vi "propagation_lbl.vi"(0 "HAS analyzer paths":T3={"Haso configuration"=path "C:/Program Files (x86)/Imagine Optic/Configuration Files/HASO4_first_7564.dat", "HAS folder"=path "N:/data/Y2019/12-Dec/19_1212/analysis/Scan026/HASOCopyAA", "subtract ref has"=FALSE, "Slopes file to subtract"=path "Z:/data/TestStand/Y2021/03-Mar/21_0303/scans/Scan006/TapeHASOCopy/Scan006_TapeHASOCopy_019.has", "Slopes file name"=path "D:/Server/10_Software/LabVIEW VIs/ImagineOptic/s35test_new.has"}, 1 "filter":T6, 2 "source wavelength [nm] (if not in has file)":dbl=800.0 format="%#_13g", 5 "Pupil":T1, 7 "Perfect lens":T10={"lens_m"=0.0, "KeepCurvature"=TRUE}, 9 "defocus":sgl, 11 "error in (no error)":errorcluster, 12 "filter":bool) -> (3 "StatisticsData":T5, 4 "PSF values":sgl[][](graph), 6 "PSF_Dimensions_um":T7, 8 "radius_mm":sgl, 10 "Wavefront (micron)":sgl[][](graph), 14 "parameters":T4, 15 "error out":errorcluster)   [LabVIEW 2020]
uses:
  WaveKit/Controls/StatisticsData.ctl
  WaveKit/Controls/SlopesPostProcessorList - Add lens.ctl
  WaveKit/Controls/General dimensions definition.ctl
  WaveKit/Controls/Point2D.ctl
  WaveKit/Controls/Point2Df.ctl
  WaveKit/Controls/HAS File information.ctl
  WaveKit/Controls/SlopesPostProcessorList - Filter.ctl
  HAS analyzer paths.ctl
  pupil ajg.ctl
  WaveKit/Classes/HasoSlopes/HasoSlopes.lvclass
  WaveKit/Classes/Pupil/Pupil.lvclass
  WaveKit/Classes/HasoField/HasoField.lvclass
  WaveKit/Classes/SurfaceFloat/SurfaceFloat.lvclass
  WaveKit/Classes/Phase/Phase.lvclass
  WaveKit/Classes/HasoData/HasoData.lvclass
  WaveKit/Classes/ComputePhaseSet/ComputePhaseSet.lvclass
panel:
  out "Zernike pupil":i32[][](graph)
  in  "PSF":bool
  out "HAS file information":T9 {"Source wavelength (nm)" format="%#_2g"}
  out "Dimension_um":T7
  in  "param":T11={"null_phase"=FALSE, "flat_intensity"=TRUE}
  out "PSF Statistics":T5={"PV"=1374189.0, "RMS"=17526034.0, "Max"=17526036.0, "Min"=1.2032529}
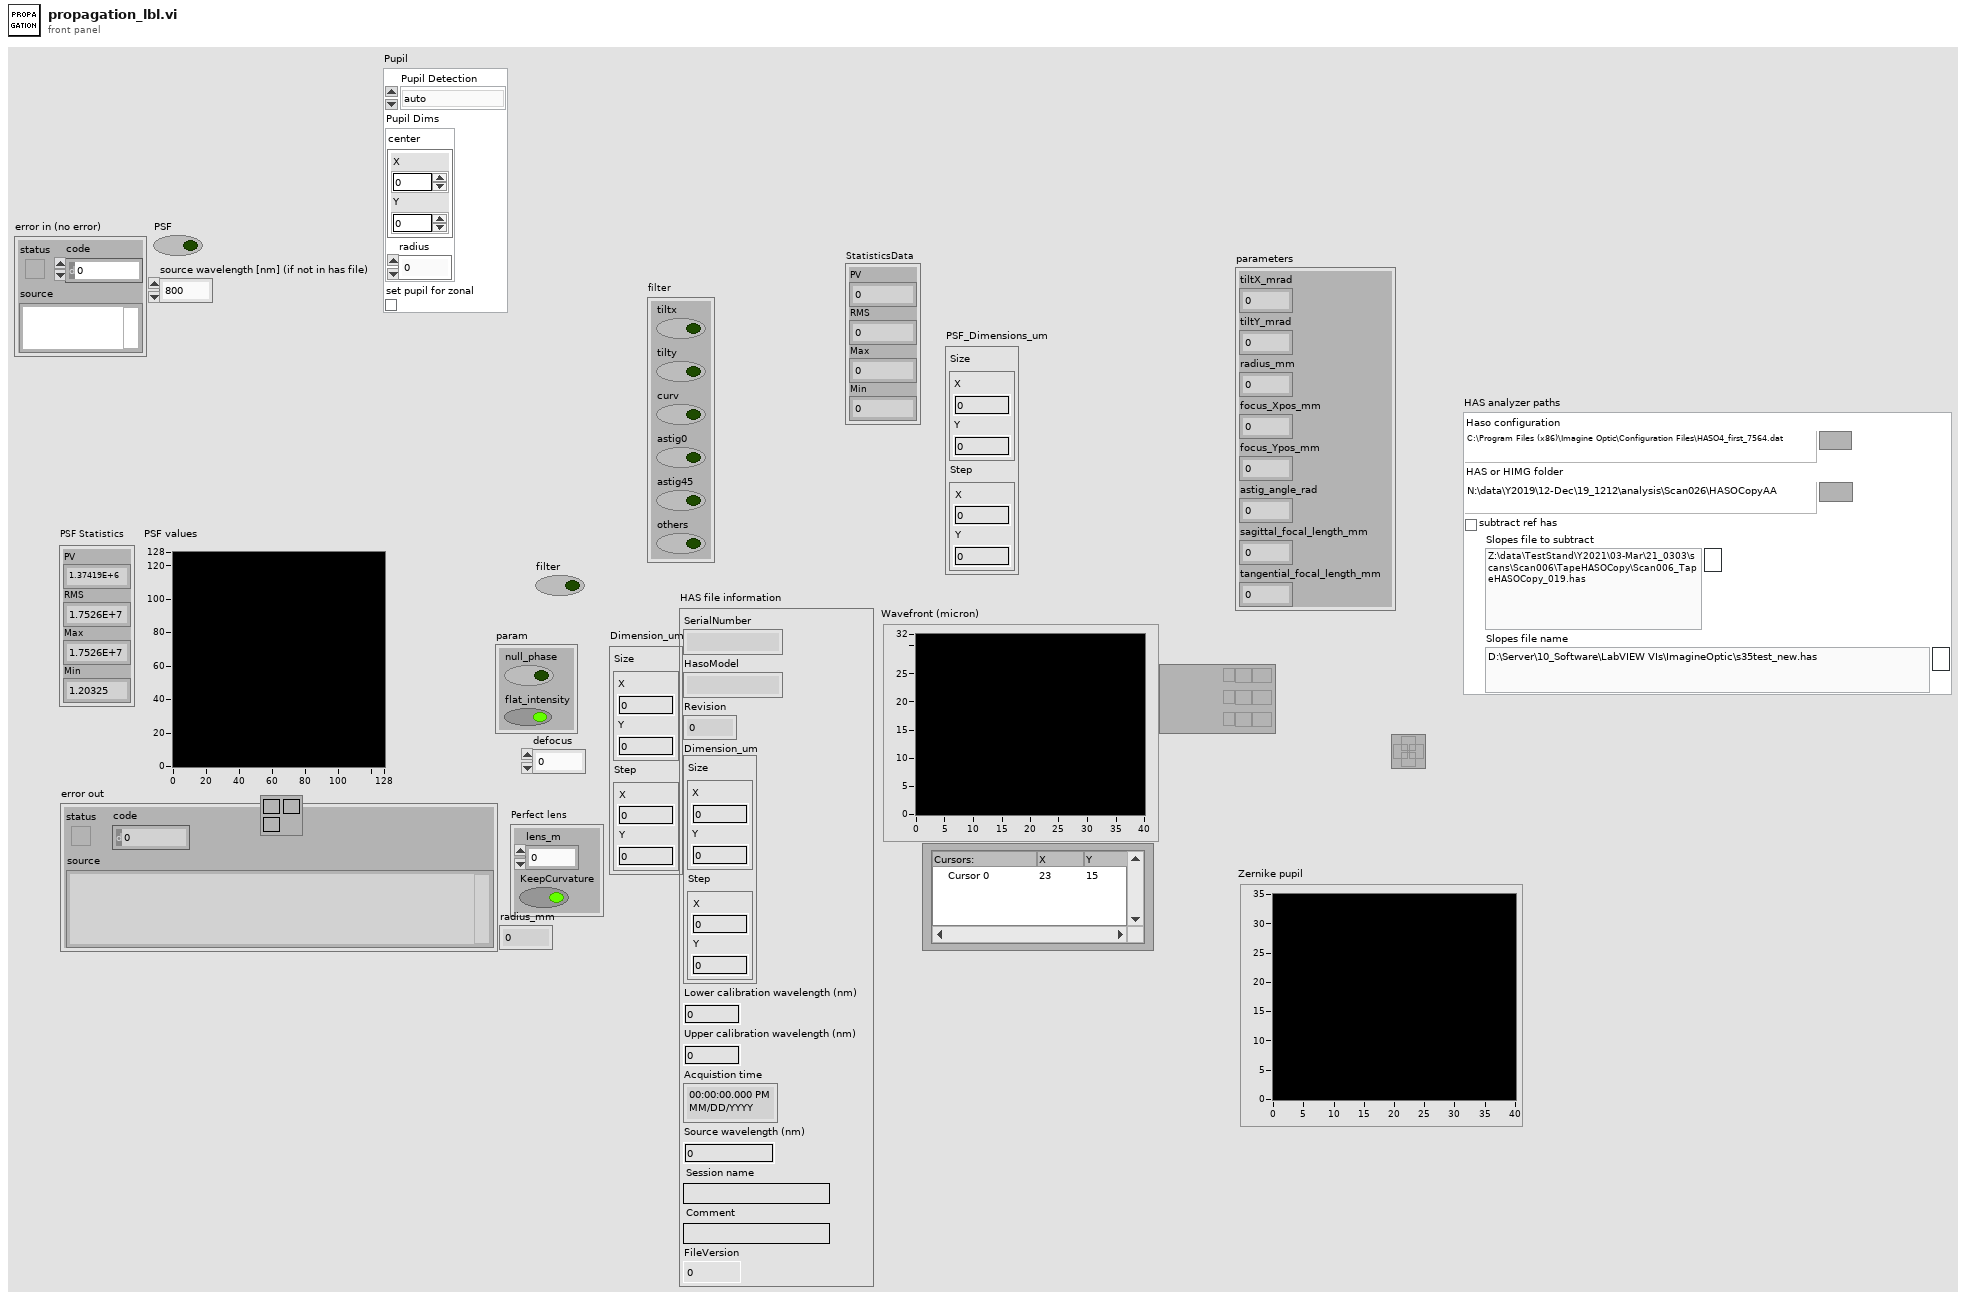
[diagram p1: front panel]
types:
  T1 = typedef "pupil ajg.ctl" = cluster{"Pupil Detection":enum16{"auto", "auto 1st shot only", "manual"}, "Pupil Dims":cluster{"center":T2, "radius":sgl}, "set pupil for zonal":bool}
  T2 = typedef "Point2Df.ctl" = cluster{"X":sgl, "Y":sgl}
  T3 = typedef "HAS analyzer paths.ctl" = cluster{"Haso configuration":path, "HAS folder":path, "subtract ref has":bool, "Slopes file to subtract":path, "Slopes file name":path}
  T4 = cluster{"tiltX_mrad":sgl, "tiltY_mrad":dbl, "radius_mm":sgl, "focus_Xpos_mm":sgl, "focus_Ypos_mm":sgl, "astig_angle_rad":sgl, "sagittal_focal_length_mm":sgl, "tangential_focal_length_mm":sgl}
  T5 = typedef "StatisticsData.ctl" = cluster{"PV":sgl, "RMS":dbl, "Max":sgl, "Min":sgl}
  T6 = typedef "SlopesPostProcessorList - Filter.ctl" = cluster{"tiltx":bool, "tilty":bool, "curv":bool, "astig0":bool, "astig45":bool, "others":bool}
  T7 = typedef "General dimensions definition.ctl" = cluster{"Size":T8, "Step":T2}
  T8 = typedef "Point2D.ctl" = cluster{"X":u32, "Y":u32}
  T9 = typedef "HAS File information.ctl" = cluster{"SerialNumber":string, "HasoModel":string, "Revision":u32, "Dimension_um":T7, "Lower calibration wavelength (nm)":dbl, "Upper calibration wavelength (nm)":dbl, "Acquistion time":timestamp, "Source wavelength (nm)":dbl, "Session name":string, "Comment":string, "FileVersion":i32}
  T10 = typedef "SlopesPostProcessorList - Add lens.ctl" = cluster{"lens_m":sgl, "KeepCurvature":bool}
  T11 = cluster{"null_phase":bool, "flat_intensity":bool}
  T12 = typedef "DataHaso acquisition information.ctl" = cluster{"HASO information":T13, "Acquisition information":T14, "SLOPES ENGINE information":T18, "Source wavelength (nm)":dbl, "FillPercent_%":dbl, "session_name":string}
  T13 = typedef "HASO information.ctl" = cluster{"HASO serial number":string, "HASO model":string, "Lower calibration wavelength (nm)":dbl, "Upper calibration wavelength (nm)":dbl, "Revision":i32}
  T14 = typedef "Image information.ctl" = cluster{"Image general information":T15, "Acquisition information":T16, "Number of pixels":T8, "Number of bits":T17}
  T15 = typedef "Image general information.ctl" = cluster{"Camera serial number":string, "Smearing removed":bool, "Background image removed":bool, "Time Stamp":timestamp, "Comment":string, "Camera_MAX_Level":i32}
  T16 = typedef "Image acquisition information.ctl" = cluster{"Exposure duration (us)":i32, "Exposure duration specified (us)":i32, "Gain":sgl, "Number of summed images":i32, "Trigger type":string}
  T17 = typedef "Data alignment enum.ctl" = enum16{"8", "16", "32"}
  T18 = typedef "SlopesEngineSetup.ctl" = cluster{"Start sub-aperture":T8, "Pupil average":dbl, "AutoStartSub-aperture":bool}
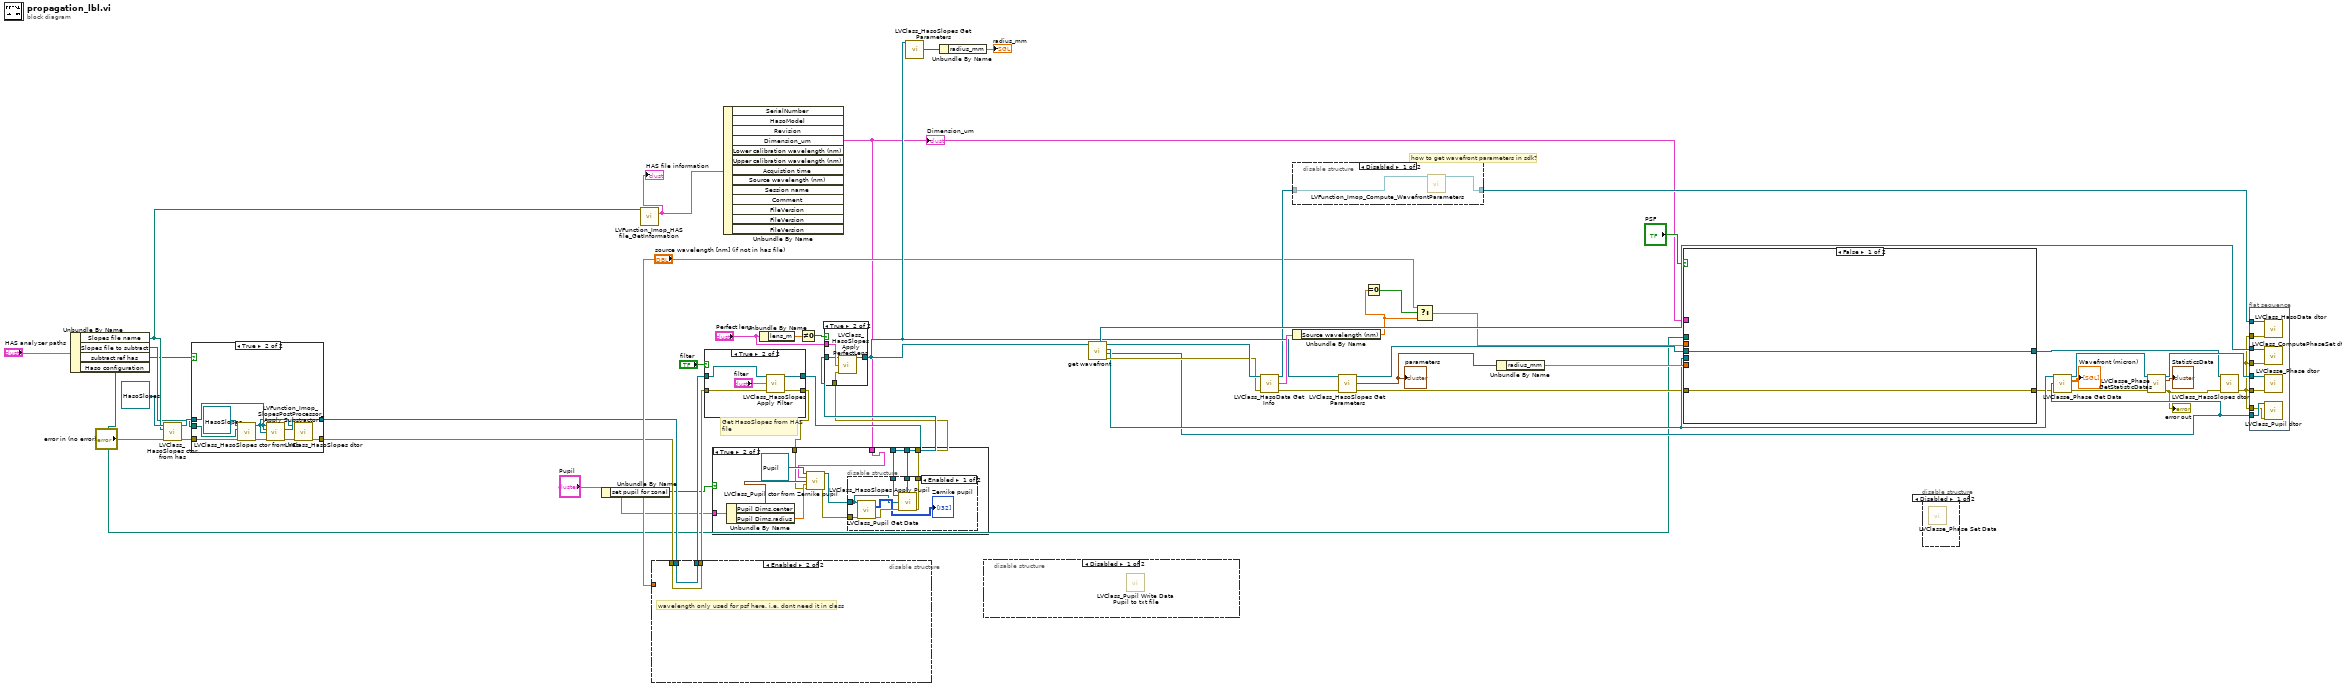
[diagram p0: block diagram]
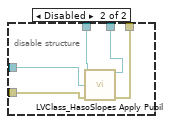
[diagram p3: hidden frame]
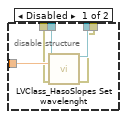
[diagram p6: hidden frame]
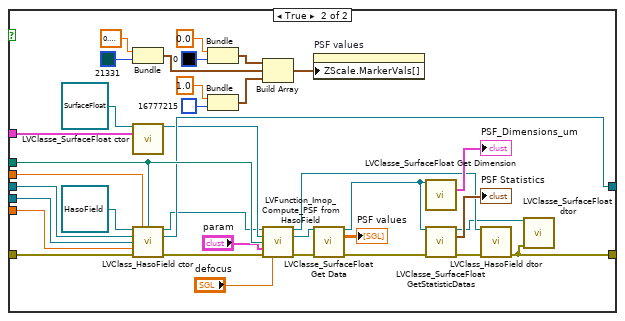
[diagram p7: hidden frame]
diagram:
  # "how to get wavefront parameters in sdk?"
  # "Get HasoSlopes from HAS file"
  n1 = Unbundle By Name("HAS analyzer paths") -> ("Slopes file name"=w10:path, "Slopes file to subtract"=w9:path, "subtract ref has"=w8:bool, "Haso configuration"=w11:path)
  n2 = call "LVClass_HasoSlopes ctor from has.vi"("HasoSlopes (const)"=refnum<class "HasoSlopes.lvclass"> refnum ("HasoSlopes in"), ".has path"=w10, "error in (no error)"="error in (no error)") -> ("HasoSlopes (new)"=w16:refnum<class "HasoSlopes.lvclass">, "error out"=w15:errorcluster)  [unwired: 11 in]
  n3 = case shown="True" w8 {
    tunnel: w9 -> [_ w66]
    tunnel: [w57 w65] -> w17
    tunnel: w16 -> [w57 w64]
    tunnel: w15 -> [w56 w63]
    tunnel: [w56 w60] -> w14
    frame False {
    }
    frame True {
      n4 = call "LVClass_HasoSlopes ctor from has.vi"("HasoSlopes (const)"=refnum<class "HasoSlopes.lvclass"> refnum ("HasoSlopes in"), ".has path"=w66, "error in (no error)"=w63) -> ("HasoSlopes (new)"=w58:refnum<class "HasoSlopes.lvclass">, "error out"=w62:errorcluster)  [unwired: 11 in]
      n5 = call "LVFunction_Imop_SlopesPostProcessor_Apply Substractor.vi"("HasoSlopes in"=w64, "HasoSlopes OUT"=w64, "HasoSlopes to substract"=w58, "error in (no error)"=w62) -> ("HasoSlopes OUT 2"=w65:refnum<class "HasoSlopes.lvclass">, "error out"=w61:errorcluster)  [unwired: 9 in, 1 out]
      n6 = call "LVClass_HasoSlopes dtor.vi"("HasoSlopes in"=w58, "error in (no error)"=w61) -> ("error out"=w60:errorcluster)  [unwired: 12 in, 1 out]
    }
  }
  n7 = Unbundle By Name("Pupil") -> ("set pupil for zonal"=w1:bool)
  n8 = call "LVFunction_Imop_HAS file_GetInformation.vi"("HAS file path"=w10) -> ("HAS file information"=w42:T9)  [unwired: 13 in, 1 out]
  "HAS file information" <- w42
  n9 = disable-structure shown="Enabled" {
    disable-tunnel: "source wavelength [nm] (if not in has file)" -> [w71 _]
    disable-tunnel: w17 -> [w70 w72]
    disable-tunnel: [w69 w72] -> w19
    disable-tunnel: w14 -> [w68 w73]
    disable-tunnel: [w67 w73] -> w18
    frame Disabled {
      n10 = call "LVClass_HasoSlopes Set wavelenght.vi"("HasoSlopes in"=w70, "Wavelenght nm"=w71, "error in (no error)"=w68) -> ("HasoSlopes out"=w69:refnum<class "HasoSlopes.lvclass">, "error out"=w67:errorcluster)  [unwired: 11 in]
    }
    frame Enabled {
      # "wavelength only used for psf here. i.e. dont need it in class"
    }
  }
  n11 = case shown="True" "filter" {
    tunnel: w19 -> [w75 w79]
    tunnel: [w75 w78] -> w5
    tunnel: w18 -> [w74 w77]
    tunnel: [w74 w76] -> w3
    frame False {
    }
    frame True {
      n12 = call "LVClass_HasoSlopes Apply Filter.vi"("HasoSlopes in"=w79, "filter"="filter", "error in (no error)"=w77) -> ("HasoSlopes out"=w78:refnum<class "HasoSlopes.lvclass">, "error out"=w76:errorcluster)  [unwired: 11 in]
    }
  }
  n13 = Unbundle By Name(w42) -> ("Dimension_um"=w4:T7)  [unwired: 12 out]
  "Dimension_um" <- w4
  n14 = case shown="True" w1 {
    tunnel: [w82 w93] -> w7
    tunnel: [w81 w89] -> w6
    tunnel: w5 -> [w82 w88]
    tunnel: w4 -> [_ w87]
    tunnel: w3 -> [w81 w84]
    tunnel: "Pupil" -> [_ w83]
    frame False {
    }
    frame True {
      n15 = Unbundle By Name(w83) -> ("Pupil Dims.center"=w86:T2, "Pupil Dims.radius"=w85:sgl)
      n16 = call "LVClass_Pupil ctor from Zernike pupil.vi"("Pupil (const)"=refnum<class "Pupil.lvclass"> refnum ("Pupil in"), "Dimensions_um"=w87, "center"=w86, "rayon"=w85, "error constant"=w84) -> ("Pupil (new)"=w91:refnum<class "Pupil.lvclass">, "error IO"=w90:errorcluster)  [unwired: 9 in]
      n17 = disable-structure shown="Enabled" {
        disable-tunnel: [w100 w103] -> w93
        disable-tunnel: w91 -> [w94 w105]
        disable-tunnel: w90 -> [w99 w102]
        disable-tunnel: [w97 w101] -> w89
        disable-tunnel: w88 -> [w96 w104]
        frame Enabled {
          n18 = call "LVClass_Pupil Get Data.vi"("Pupil in"=w94, "error in (no error)"=w99) -> ("Data"=→"Zernike pupil":i32[][], "error out"=w98:errorcluster)  [unwired: 11 in, 1 out]
          n19 = call "LVClass_HasoSlopes Apply Pupil.vi"("HasoSlopes in"=w96, "Pupil IN"=w94, "error in (no error)"=w98) -> ("HasoSlopes out"=w100:refnum<class "HasoSlopes.lvclass">, "error out"=w97:errorcluster)  [unwired: 11 in]
        }
        frame Disabled {
          n20 = call "LVClass_HasoSlopes Apply Pupil.vi"("HasoSlopes in"=w104, "Pupil IN"=w105, "error in (no error)"=w102) -> ("HasoSlopes out"=w103:refnum<class "HasoSlopes.lvclass">, "error out"=w101:errorcluster)  [unwired: 11 in]
        }
      }
    }
  }
  n21 = Unbundle By Name("Perfect lens") -> ("lens_m"=w45:sgl)
  n22 = Not Equal To 0?(x=w45) -> (x != 0?=w44:bool)
  n23 = case shown="True" w44 {
    tunnel: [w106 w110] -> w41
    tunnel: w7 -> [w106 w108]
    tunnel: "Perfect lens" -> [_ w109]
    tunnel: w6 -> [_ w107]
    frame False {
    }
    frame True {
      n24 = call "LVClass_HasoSlopes Apply PerfectLens.vi"("HasoSlopes in"=w108, "Perfect lens"=w109, "error in (no error)"=w107) -> ("HasoSlopes out"=w110:refnum<class "HasoSlopes.lvclass">)  [unwired: 11 in, 1 out]
    }
  }
  n25 = call "LVClass_HasoSlopes Get Parameters.vi"("HasoSlopes in"=w41) -> ("Pamameter"=w40:T4)  [unwired: 12 in, 2 out]
  n26 = Unbundle By Name(w40) -> ("radius_mm"=→"radius_mm":sgl)
  n27 = disable-structure shown="Disabled" {
    frame Disabled {
      n28 = call "LVClass_Pupil Write Data Pupil to txt file.vi"() -> ()  [unwired: 14 in, 2 out]
    }
    frame Enabled {
    }
  }
  n29 = call "get wavefront.vi"("HasoSlopes in"=w41) -> ("error out"=w48:errorcluster, "Pupil (new)"=w37:refnum<class "Pupil.lvclass">, "Phase"=w38:refnum<class "Phase.lvclass">, "HasoData out"=w50:refnum<class "HasoData.lvclass">, "ComputePhaseSet.lvclass 2"=w49:refnum<class "ComputePhaseSet.lvclass">)  [unwired: 6 in]
  n30 = call "LVClass_HasoData Get Info.vi"("HasoData in"=w50, "error in (no error)"=w48) -> ("HasoData out"=w31:refnum<class "HasoData.lvclass">, "DataHaso acquisition information"=w52:T12, "error out"=w51:errorcluster)  [unwired: 11 in]
  n31 = disable-structure shown="Disabled" {
    disable-tunnel: w31 -> [w112 w113]
    disable-tunnel: [w111 w113] -> w30
    frame Disabled {
      n32 = call "LVFunction_Imop_Compute_WavefrontParameters.vi"("HasoData.lvclass"=w112) -> ("HasoData.lvclass (dup)"=w111:refnum<class "HasoData.lvclass">)  [unwired: 12 in, 2 out]
    }
    frame Enabled {
    }
  }
  n33 = Unbundle By Name(w52) -> ("Source wavelength (nm)"=w21:dbl)
  n34 = call "LVClass_HasoSlopes Get Parameters.vi"("HasoSlopes in"=w41, "error in (no error)"=w51) -> ("HasoSlopes out"=w54:refnum<class "HasoSlopes.lvclass">, "Pamameter"=w29:T4, "error out"=w12:errorcluster)  [unwired: 11 in]
  "parameters" <- w29
  n35 = Equal To 0?(x=w21) -> (x = 0?=w47:bool)
  n36 = Select(t="source wavelength [nm] (if not in has file)", s=w47, f=w21) -> (s? t:f=w46:dbl)
  n37 = Unbundle By Name(w29) -> ("radius_mm"=w53:sgl)
  n38 = case shown="False" "PSF" {
    tunnel: w54 -> [w115 w151]
    tunnel: w53 -> [_ w150]
    tunnel: w46 -> [_ w149]
    tunnel: w4 -> [_ w148]
    tunnel: w11 -> [_ w147]
    tunnel: w38 -> [_ w146]
    tunnel: w12 -> [w114 w145]
    tunnel: [w115 w144] -> w27
    tunnel: [w114 w143] -> w24
    frame False {
    }
    frame True {
      n39 = Bundle(sgl 0.2, u32 21331) -> (w125:cluster{sgl, u32})  [unwired: 1 in]
      n40 = call "LVClasse_SurfaceFloat ctor.vi"("SurfaceFloat (const)"=refnum<class "SurfaceFloat.lvclass"> refnum ("SurfaceFloat in"), "Dimensions_um"=w148) -> ("SurfaceFloat (new)"=w142:refnum<class "SurfaceFloat.lvclass">)  [unwired: 12 in, 1 out]
      n41 = call "LVClass_HasoField ctor.vi"("HasoField (const)"=refnum<class "HasoField.lvclass"> refnum ("HasoField in"), "wavelenght nm"=w149, "haso_config_file_path"=w147, "HasoSlopes"=w151, "Phase"=w146, "radius_of_curvature _ mm"=w150, "error in (no error)"=w145) -> ("HasoField (new)"=w132:refnum<class "HasoField.lvclass">, "HasoSlopes (dup)"=w144:refnum<class "HasoSlopes.lvclass">, "error out"=w128:errorcluster)  [unwired: 4 in, 2 out]
      n42 = Bundle(0.0, u32 0) -> (w122:cluster{dbl, u32})  [unwired: 1 in]
      n43 = Bundle(sgl 1.0, u32 16777215) -> (w124:cluster{sgl, u32})  [unwired: 1 in]
      n44 = Build Array(w122, w125, w124) -> (w123:cluster{dbl, u32}[])
      n45 = call "LVFunction_Imop_Compute_PSF from HasoField.vi"("HasoField in"=w132, "Surface PSF"=w142, "Path"=w147, "param"="param", "error in (no error)"=w128, "defocus"="defocus") -> ("HasoField out"=w127:refnum<class "HasoField.lvclass">, "Surface PSF"=w137:refnum<class "SurfaceFloat.lvclass">, "error out"=w136:errorcluster)  [unwired: 7 in]
      n46 = property on="PSF values" class="IntGraph (strict)"("ZScale.MarkerVals[]"=w123) -> ()  [unwired: 2 in, 2 out]
      n47 = call "LVClasse_SurfaceFloat Get Data.vi"("SurfaceFloat in"=w137, "error in (no error)"=w136) -> ("SurfaceFloat out"=w129:refnum<class "SurfaceFloat.lvclass">, "data"=→"PSF values":sgl[][], "error out"=w139:errorcluster)  [unwired: 11 in]
      n48 = call "LVClasse_SurfaceFloat Get Dimension.vi"("SurfaceFloat in"=w129) -> ("Dimensions_um"=→"PSF_Dimensions_um":T7)  [unwired: 12 in, 2 out]
      n49 = call "LVClasse_SurfaceFloat GetStatisticDatas.vi"("SurfaceFloat in"=w129, "error in (no error)"=w139) -> ("SurfaceFloat out"=w126:refnum<class "SurfaceFloat.lvclass">, "StatisticsData"=→"PSF Statistics":T5, "error out"=w135:errorcluster)  [unwired: 11 in]
      n50 = call "LVClass_HasoField dtor.vi"("HasoField in"=w127, "error in (no error)"=w135) -> ("error out"=w143:errorcluster)  [unwired: 12 in, 1 out]
      n51 = call "LVClasse_SurfaceFloat dtor.vi"("SurfaceFloat in"=w126, "error in (no error)"=w143) -> ()  [unwired: 12 in, 2 out]
    }
  }
  n52 = disable-structure shown="Disabled" {
    frame Disabled {
      n53 = call "LVClasse_Phase Set Data.vi"() -> ()  [unwired: 14 in, 2 out]
    }
    frame Enabled {
    }
  }
  n54 = call "LVClasse_Phase Get Data.vi"("Phase in"=w38, "Pupil"=w37, "error in (no error)"=w24) -> ("Phase out"=w34:refnum<class "Phase.lvclass">, "data"=→"Wavefront (micron)":sgl[][], "error out"=w23:errorcluster)  [unwired: 9 in, 1 out]
  n55 = call "LVClasse_Phase GetStatisticDatas.vi"("Phase in"=w34, "error in (no error)"=w23) -> ("Phase out"=w33:refnum<class "Phase.lvclass">, "StatisticsData"=→"StatisticsData":T5, "error out"=w22:errorcluster)  [unwired: 11 in]
  "error out" <- w22
  n56 = call "LVClass_HasoSlopes dtor.vi"("HasoSlopes in"=w27, "error in (no error)"=w22) -> ("error out"=w25:errorcluster)  [unwired: 12 in, 1 out]
  n57 = flat-sequence {
    tunnel: w49 -> [w159]
    tunnel: w30 -> [w158]
    tunnel: w37 -> [w157]
    tunnel: w25 -> [w156]
    tunnel: w25 -> [w155]
    tunnel: w25 -> [w154]
    tunnel: w25 -> [w153]
    tunnel: w33 -> [w152]
    frame #0 {
      n58 = call "LVClass_HasoData dtor.vi"("HasoData in"=w158, "error in (no error)"=w154) -> ()  [unwired: 12 in, 2 out]
      n59 = call "LVClass_ComputePhaseSet dtor.vi"("ComputePhaseSet in"=w159, "error in (no error)"=w153) -> ()  [unwired: 12 in, 2 out]
      n60 = call "LVClasse_Phase dtor.vi"("Phase in"=w152, "error in (no error)"=w155) -> ()  [unwired: 12 in, 2 out]
      n61 = call "LVClass_Pupil dtor.vi"("Pupil in"=w157, "error in (no error)"=w156) -> ()  [unwired: 12 in, 2 out]
    }
  }
